vi "Init.vi"(8 "error in (no error)":errorcluster, 11 "DB Path":path) -> (0 "error out":errorcluster, 3 "Config-Sqlite out":refnum<class "Config-Sqlite.lvclass">)   [LabVIEW 2020, in "CDM-Config.lvlib" / "Config-Sqlite.lvclass"]
doc: "Creates a SQLite storage instance capable of saving to and loading from a SQLite db file. Storage is done in two tables, one for the elements where each row is a single element and a second table for the meta fields linked back to the owning element row."
uses:
  Config-Sqlite.lvclass
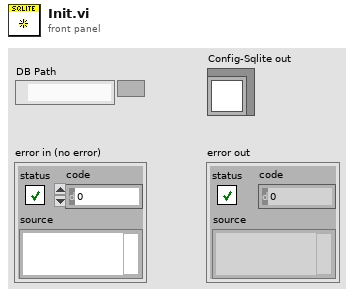
[diagram p1: front panel]
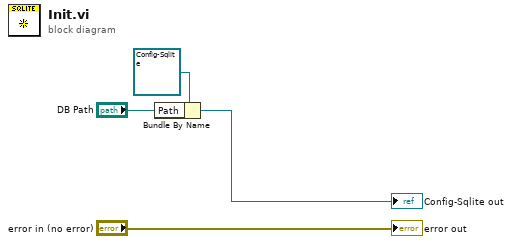
[diagram p0: block diagram]
diagram:
  n1 = Bundle By Name(cluster=refnum<class "Config-Sqlite.lvclass"> refnum ("Config-Sqlite in"), "Path"="DB Path") -> (→"Config-Sqlite out":refnum<class "Config-Sqlite.lvclass">)
  "error out" <- "error in (no error)"
